vi "Save_Truth_Table.vi"(8 "Stop":bool, 9 "first iteration":bool, 10 "Timeout 2":bool, 11 "Timeout 1":bool) -> (1 "Append Sample Data 2":bool, 2 "Save_Data":bool, 3 "Append Sample Data 1":bool)   [LabVIEW 2024]
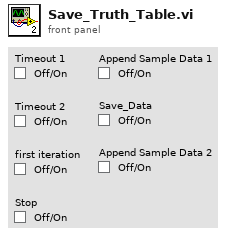
[diagram p1: front panel]
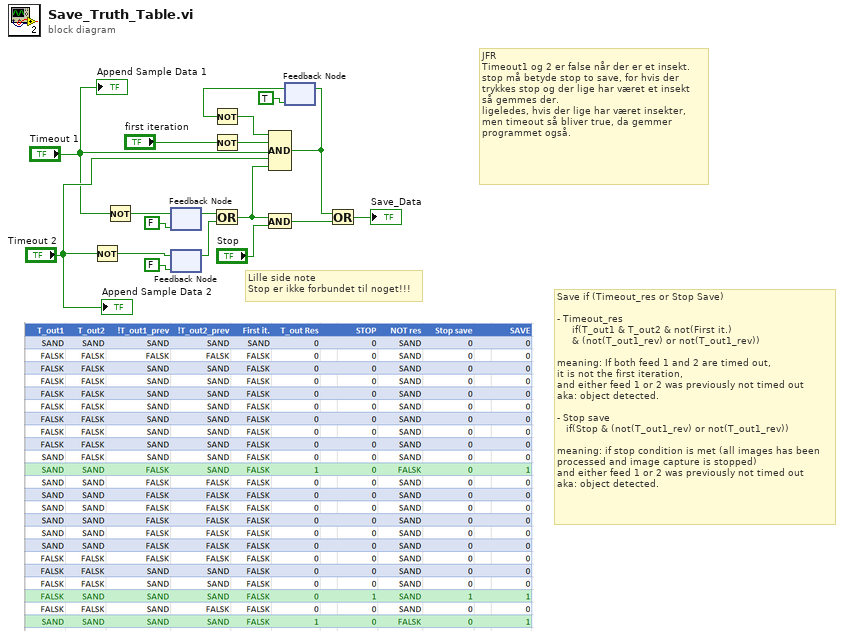
[diagram p0: block diagram]
diagram:
  # "Lille side note\nStop er ikke forbundet til noget!!!"
  # "JFR\nTimeout1 og 2 er false når der er et insekt.\nstop må betyde stop to save, for hvis der \ntrykkes stop og der lige har været et insekt \nså gemmes der. \nligeledes, hvis der lige har været insekter, \nmen timeout så bliver true, da gemmer \nprogrammet også."
  # "Save if (Timeout_res or Stop Save)\n\n- Timeout_res\n     if(T_out1 & T_out2 & not(First it.) \n     & (not(T_out1_rev) or not(T_out1_rev))\n\nmeaning: If both feed 1 and 2 are timed out,\nit is not the first iteration,\nand either feed 1 or 2 was previously not timed out\naka: object detected.\n\n- Stop save\n   if(Stop & (not(T_out1_rev) or not(T_out1_rev))\n\nmeaning: if stop condition is met (all images has been\nprocessed and image capture is stopped)\nand either feed 1 or 2 was previously not timed out\naka: object detected."
  n1 = Not(x="Timeout 2") -> (.not. x?=w1:bool)
  n2 = Not(x="Timeout 1") -> (.not. x?=w2:bool)
  n3 = feedback #1(FALSE ("Timeout 2")) -> (w6:bool)
  n4 = feedback-in #1(w2) -> ()
  n5 = feedback #2(FALSE ("Timeout 2")) -> (w7:bool)
  n6 = feedback-in #2(w1) -> ()
  n7 = Not(x="first iteration") -> (.not. x?=w4:bool)
  n8 = Or(x=w6, y=w7) -> (x .or. y?=w13:bool)
  n9 = And(x=w13, y="Stop") -> (x .and. y?=w16:bool)
  n10 = feedback #3(TRUE) -> (w8:bool)
  n11 = Not(x=w8) -> (.not. x?=w5:bool)
  n12 = Compound Arithmetic op=AND(w5, w4, "Timeout 1", "Timeout 2", w13) -> (w14:bool)
  n13 = feedback-in #3(w14) -> ()
  n14 = Or(x=w14, y=w16) -> (x .or. y?=→"Save_Data":bool)
  "Append Sample Data 2" <- "Timeout 2"
  "Append Sample Data 1" <- "Timeout 1"
